vi "Or77200_GPIB_VisaRW.vi"() -> ()   [LabVIEW 2010]
panel:
  in  "Write":bool
  in  "Use LF-Cr":bool
  in  "termination char\n(0xA = '\\n' = LF)":u8=10
  in  "Serial Settings:Stop Bits":u16(ring)=10 items=["1.0"=10, "1.5"=15, "2.0"=20]
  out "Serial Settings:Parity":u16(ring) items=["None", "Odd", "Even", "Mark", "Space"]
  in  "Serial Settings:Data Bits":u16
  in  "Serial Settings:Baud Rate":u32
  out "Port Out":refnum<visa-resource-name>
  out "ByteRead":u32
  out "Response":string
  in  "ByteToRd":u32
  out "ByteWr":u32
  in  "Commande":string
  in  "Port":refnum<visa-resource-name>
  out "error out":errorcluster
  in  "error in":errorcluster
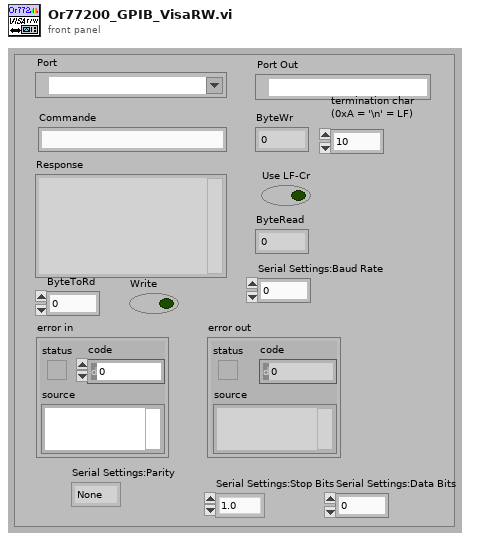
[diagram p1: front panel]
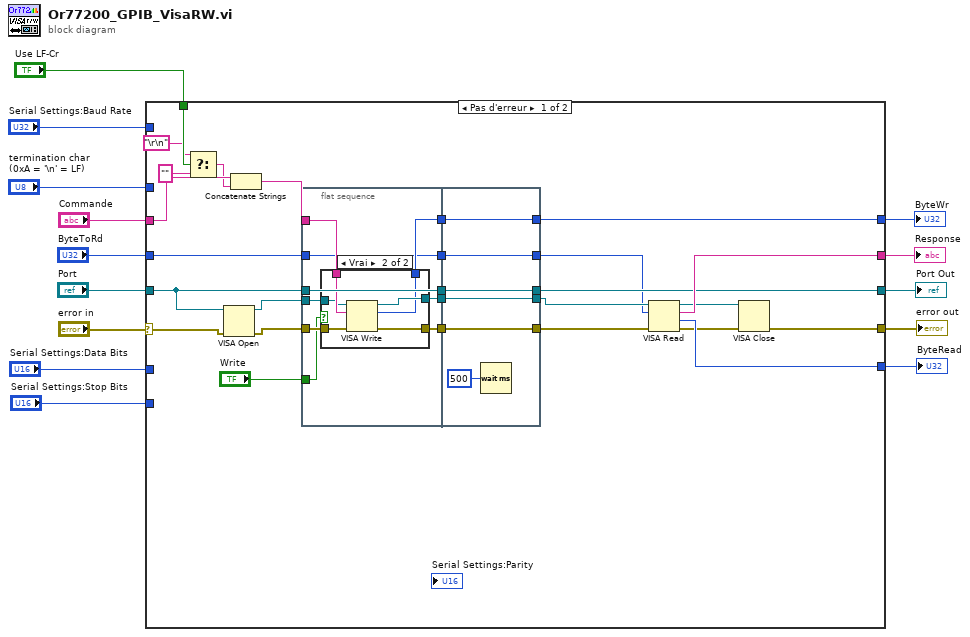
[diagram p0: block diagram]
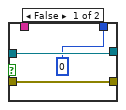
[diagram p2: hidden frame]
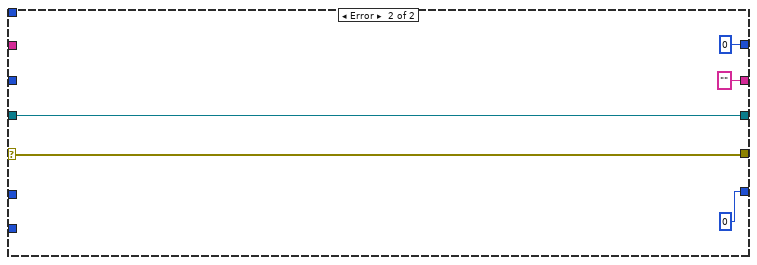
[diagram p3: hidden frame]
diagram:
  n1 = case shown="Pas d'erreur" "error in" {
    selector: "error in" -> [w25 w67]
    tunnel: "Port" -> [w23 w70]
    tunnel: "Commande" -> [w31 _]
    tunnel: [w41 u32 0 ("return count")] -> w11
    tunnel: "ByteToRd" -> [w32 _]
    tunnel: [w40 "" ("read buffer")] -> w9
    tunnel: [w20 w67] -> w8
    tunnel: [w39 u32 0 ("return count")] -> w7
    tunnel: [w35 w70] -> w6
    tunnel: "Serial Settings:Data Bits" -> [_ _]
    tunnel: "Serial Settings:Stop Bits" -> [_ _]
    tunnel: "termination char\n(0xA = '\\n' = LF)" -> [_ _]
    tunnel: "Serial Settings:Baud Rate" -> [_ _]
    tunnel: "Use LF-Cr" -> [w29 _]
    frame No Error {
      n2 = Select(t="\r\n", s=w29, f="" ("cas faux")) -> (s? t:f=w26:string)
      n3 = VISA Open(error in (no error)=w25, VISA resource name=w23) -> (VISA resource name=w22:refnum<visa-resource-name>, error out=w24:errorcluster)  [unwired: 3 in]
      n4 = Concatenate Strings(w31, w26) -> (w30:string)
      n5 = flat-sequence {
        tunnel: w30 -> [w47]
        tunnel: [w50] -> w38
        tunnel: [w49] -> w37
        tunnel: [w48] -> w36
        tunnel: w23 -> [w46]
        tunnel: [w46] -> w34
        tunnel: [w45] -> w33
        tunnel: w32 -> [w45]
        tunnel: w24 -> [w44]
        tunnel: w22 -> [w43]
        tunnel: "Write" -> [w42]
        tunnel: [w64] -> w41
        tunnel: [w65] -> w18
        tunnel: w38 -> [w60]
        tunnel: w37 -> [w65]
        tunnel: w36 -> [w64]
        tunnel: [w63] -> w35
        tunnel: w34 -> [w63]
        tunnel: [w62] -> w15
        tunnel: w33 -> [w62]
        tunnel: [w60] -> w17
        frame #0 {
          n6 = case shown="Vrai" w42 {
            tunnel: [w52 w59] -> w50
            tunnel: [w53 w58] -> w49
            tunnel: [u32 0 ("return count") w57] -> w48
            tunnel: w47 -> [_ w56]
            tunnel: w44 -> [w52 w55]
            tunnel: w43 -> [w53 w54]
            frame False {
            }
            frame True {
              n7 = VISA Write(VISA resource name=w54, write buffer=w56, error in (no error)=w55) -> (VISA resource name out=w58:refnum<visa-resource-name>, return count=w57:u32, error out=w59:errorcluster)
            }
          }
        }
        frame #1 {
          n8 = Wait (ms)(milliseconds to wait=u32 500 ("attente (ms)")) -> ()  [unwired: 1 out]
        }
      }
      n9 = VISA Read(VISA resource name=w18, byte count=w15, error in (no error)=w17) -> (VISA resource name out=w19:refnum<visa-resource-name>, read buffer=w40:string, return count=w39:u32, error out=w21:errorcluster)
      n10 = VISA Close(VISA resource name=w19, error in (no error)=w21) -> (error out=w20:errorcluster)
    }
    frame Error {
    }
  }
  "error out" <- w8
  "ByteWr" <- w11
  "Response" <- w9
  "ByteRead" <- w7
  "Port Out" <- w6
